vi "SEQ Set.vi"(8 "error in (no error)":errorcluster, 10 "dummy":bool, 11 "Data Refnum":T1) -> (0 "error out":errorcluster, 3 "Data Refnum out":T1)   [LabVIEW 2009]
doc: "This is a template VI for the SEQ Set function. It is not used in the course because the Set and Get are created with a different method that leverages scripting. \n\nAAL 9/09"
uses:
  Controls/SEQ DataRef.ctl
  Controls/SEQ Data.ctl
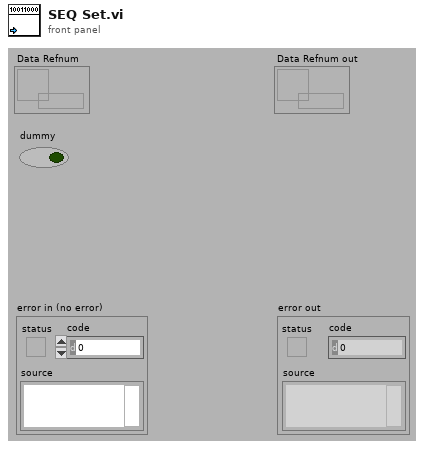
[diagram p1: front panel]
types:
  T1 = typedef "SEQ DataRef.ctl" = refnum<queue>
  T2 = typedef "SEQ Data.ctl" = cluster{"Numeric":dbl}
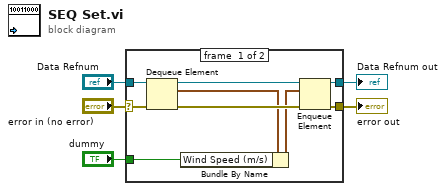
[diagram p0: block diagram]
diagram:
  n1 = case shown="No Error" "error in (no error)" {
    selector: "error in (no error)" -> [w9 w15]
    tunnel: "Data Refnum" -> [w14 w16]
    tunnel: [w11 w15] -> w4
    tunnel: [w10 w16] -> w3
    tunnel: "dummy" -> [w7 _]
    frame #0 {
      n2 = Dequeue Element(queue=w14, error in (no error)=w9) -> (queue out=w12:T1, element=w8:T2, error out=w13:errorcluster)  [unwired: 2 out]
      n3 = Bundle By Name(cluster=w8, "Wind Speed (m/s)"=w7) -> (w6:T2)
      n4 = Enqueue Element(queue=w12, element=w6, error in (no error)=w13) -> (queue out=w10:T1, error out=w11:errorcluster)  [unwired: 2 out]
    }
    frame #1 {
    }
  }
  "Data Refnum out" <- w3
  "error out" <- w4
